vi "Get or Add Sheet.vi"(8 "error in":errorcluster, 10 "Sheet Name":string, 11 "SpreadsheetDoc in":refnum<k24>) -> (0 "error out":errorcluster, 1 "Sheet Index":i32, 2 "Sheet":refnum<k24>, 3 "SpreadsheetDoc out":refnum<k24>, 5 "SheetName":string)   [LabVIEW 2019, in "Open Xml.lvlib"]
uses:
  Open Xml.lvlib
  D:/git/Open-Xml-LabVIEW/Source/DocumentFormat.OpenXml.dll
  DocumentFormat.OpenXml.dll
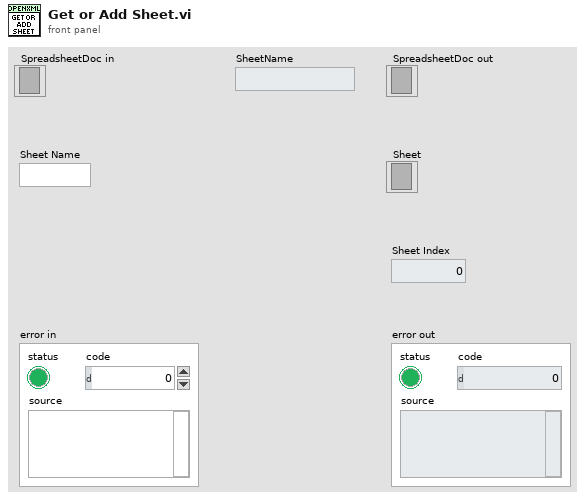
[diagram p1: front panel]
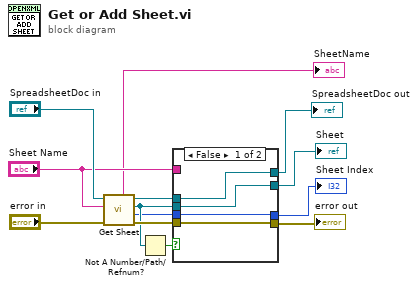
[diagram p0: block diagram]
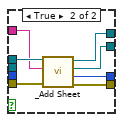
[diagram p2: hidden frame]
diagram:
  n1 = call "Get Sheet.vi"("error in"="error in", "SheetName"="Sheet Name", "SpreadsheetDoc in"="SpreadsheetDoc in") -> ("error out"=w12:errorcluster, "Sheet Index"=w1:i32, "Sheet"=w8:refnum<k24>, "SpreadsheetDoc out"=w7:refnum<k24>, "SheetName"=→"SheetName":string)  [unwired: 4 in]
  n2 = Not A Number/Path/Refnum?(number/path/refnum=w8) -> (NaN/Path/Refnum?=w9:bool)
  n3 = case shown="False" w9 {
    tunnel: [w15 w24] -> w13
    tunnel: w12 -> [w15 w23]
    tunnel: w8 -> [w17 _]
    tunnel: w7 -> [w16 w22]
    tunnel: [w16 w21] -> w6
    tunnel: "Sheet Name" -> [_ w20]
    tunnel: [w17 w19] -> w4
    tunnel: [w14 w18] -> w2
    tunnel: w1 -> [w14 _]
    frame False {
    }
    frame True {
      n4 = call "_Add Sheet.vi"("error in"=w23, "SheetName"=w20, "SpreadsheetDoc in"=w22) -> ("error out"=w24:errorcluster, "Sheet Index"=w18:i32, "Sheet"=w19:refnum<k24>, "SpreadsheetDoc out"=w21:refnum<k24>)  [unwired: 5 in]
    }
  }
  "error out" <- w13
  "Sheet" <- w4
  "SpreadsheetDoc out" <- w6
  "Sheet Index" <- w2
